vi "Remove App.vi"(8 "error in (no error)":errorcluster, 10 "App":refnum<class "ViaApp.lvclass">, 11 "App Watcher in":refnum<class "App Watcher.lvclass">) -> (0 "error out":errorcluster, 3 "App Watcher out":refnum<class "App Watcher.lvclass">)   [LabVIEW 2020, in "PicoG-App.lvlib" / "App Watcher.lvclass"]
uses:
  App Watcher.lvclass
  ViaApp/ViaApp.lvclass
  App Watcher.lvclass/App Watcher.ctl
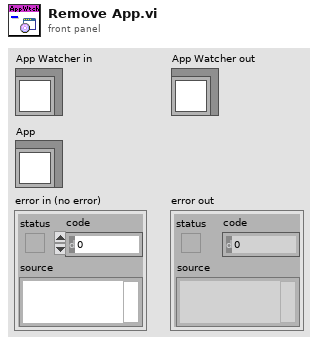
[diagram p1: front panel]
types:
  T1 = typedef "PicoG-App.lvlib/App Watcher.lvclass/Ref Data.ctl" = cluster{"App Map":map{path, refnum<class "ViaApp.lvclass">}, "App Update Event":refnum<user-event>}
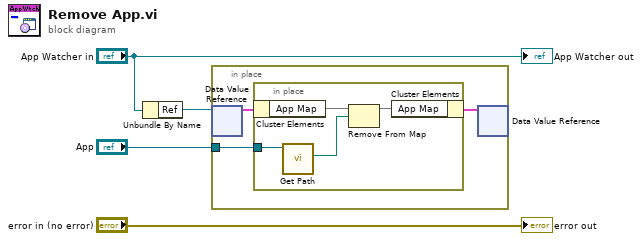
[diagram p0: block diagram]
diagram:
  n1 = Unbundle By Name("App Watcher in") -> ("Ref"=w3:refnum<data-value>)
  n2 = in-place {
    in-place-border: "App" -> [w5]
    n3 = in-place-dvr #1(w3) -> (w7:T1)  [unwired: 1 out]
    n4 = in-place {
      in-place-border: w5 -> [w11]
      n5 = in-place-cluster #2(w7) -> ("App Map"=w10:map{path, refnum<class "ViaApp.lvclass">})
      n6 = call "Get Path.vi"("ViaApp in"=w11) -> ("Path"=w9:path)  [unwired: 8 in, 2 out]
      n7 = Remove From Map(10:w9, 11:w10) -> (3:w8:map{path, refnum<class "ViaApp.lvclass">})  [unwired: 2 out]
      n8 = in-place-cluster #2("App Map"=w8) -> (w6:T1)
    }
    n9 = in-place-dvr #1(w6) -> ()  [unwired: 2 out]
  }
  "error out" <- "error in (no error)"
  "App Watcher out" <- "App Watcher in"
